vi "Parse CRC_MAP File.vi"(8 "error in":errorcluster, 11 "file (use dialog)":path) -> (0 "error out":errorcluster, 1 "Data IDs":string[](array[string]), 2 "Msg IDs":string[](array[string]), 3 "File String Out":string)   [LabVIEW 2023, in "LP_CRC.lvlib"]
uses:
  LP_CRC.lvlib
  <vilib>/Utility/SystemLogging/NI_SystemLogging.lvlib
  <vilib>/NI VeriStand/Custom Device Tools/Custom Device Utility Library/Custom Device Utility Library.lvlib
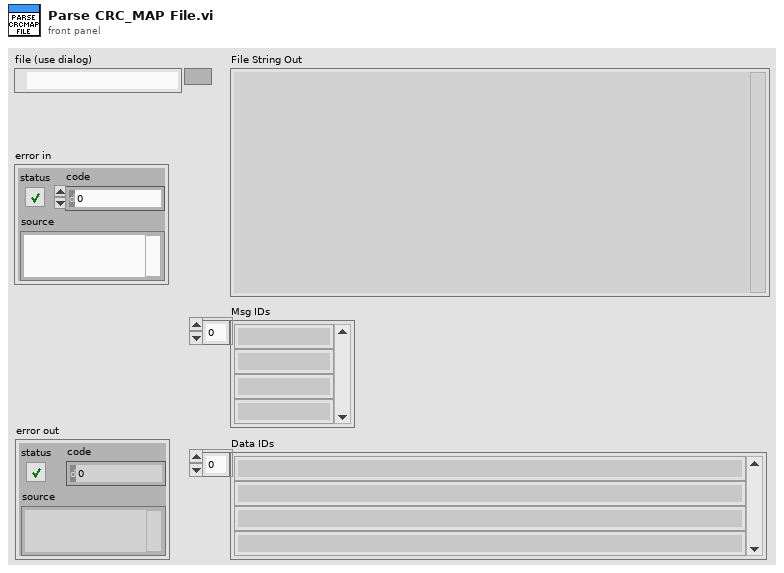
[diagram p1: front panel]
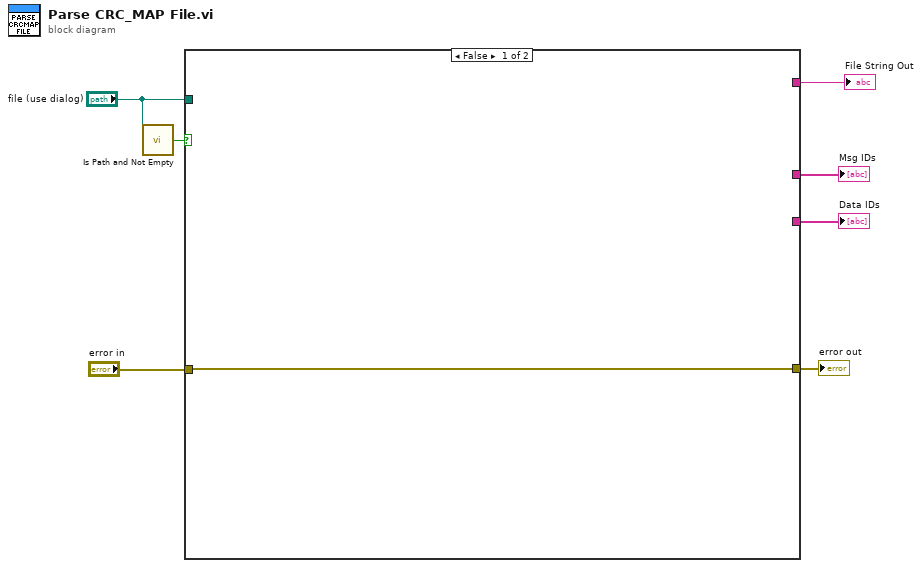
[diagram p0: block diagram]
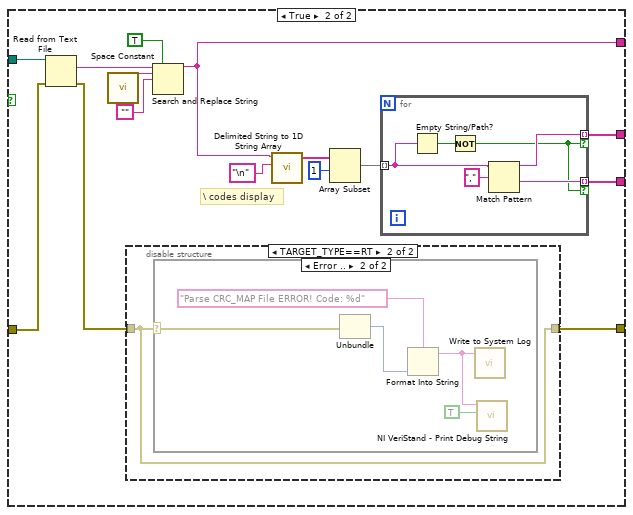
[diagram p2: hidden frame]
diagram:
  n1 = call <vilib>:"Is Path and Not Empty.vi"("path"="file (use dialog)") -> ("Is Path and Not Empty?"=w1:bool)  [unwired: 4 in]
  n2 = case shown="False" w1 {
    tunnel: [_ w20] -> w7
    tunnel: [_ w18] -> w6
    tunnel: [_ w17] -> w5
    tunnel: "error in" -> [w8 w12]
    tunnel: [w8 w11] -> w3
    tunnel: "file (use dialog)" -> [_ w9]
    frame False {
    }
    frame True {
      # "\\ codes display"
      n3 = Read from Text File(file (use dialog)=w9, error in=w12) -> (text=w23:string, error out=w13:errorcluster)  [unwired: 1 in, 3 out]
      n4 = call <vilib>:"Space Constant.vi"() -> ("String"=w21:string)
      n5 = disable-structure shown="TARGET_TYPE==RT" {
        disable-tunnel: w13 -> [w24 w25]
        disable-tunnel: [w24 w25] -> w11
        frame condition #0 (active) {
        }
        frame condition #1 {
          n6 = case shown="Error .." w25 {
            selector: w25 -> [_ w30]
            frame No Error {
            }
            frame Error {
              n7 = Unbundle(w30) -> ("code"=w29:i32)  [unwired: 2 out]
              n8 = Format Into String(format string="Parse CRC_MAP File ERROR! Code: %d", w29) -> (resulting string=w27:string)  [unwired: 2 in, 1 out]
              n9 = call <vilib>:"Write to System Log.vi"("message"=w27) -> ()  [unwired: 10 in, 1 out]
              n10 = call <vilib>:"NI VeriStand - Print Debug String.vi"("Add to log file? (F)"=TRUE, "Message"=w27) -> ()  [unwired: 9 in, 1 out]
            }
          }
        }
      }
      n11 = Search and Replace String(replace all?=TRUE ("replace all? (F)"), input string=w23, search string=w21, replace string="") -> (result string=w20:string)  [unwired: 4 in, 3 out]
      n12 = call <vilib>:"Delimited String to 1D String Array.vi"("delimiter"="\n", "delimited string"=w20) -> ("string array"=w16:string[])  [unwired: 9 in]
      n13 = Array Subset(array=w16, index=1) -> (w15:string[])  [unwired: 1 in]
      n14 = for {
        tunnel: w15 -> [w33] mode=indexing
        tunnel: [w36] -> w18 mode=indexing if=w31
        tunnel: [w34] -> w17 mode=indexing if=w31
        n15 = Empty String/Path?(string/path=w33) -> (empty?=w32:bool)
        n16 = Not(x=w32) -> (.not. x?=w31:bool)
        n17 = Match Pattern(string=w33, regular expression=",") -> (before substring=w36:string, after substring=w34:string)  [unwired: 1 in, 2 out]
      }
    }
  }
  "File String Out" <- w7
  "Msg IDs" <- w6
  "Data IDs" <- w5
  "error out" <- w3
